vi "sc_decode.vi"(1 "SC_bits":dbl[](array[numeric])) -> (0 "Place opened":string)   [LabVIEW 2017]
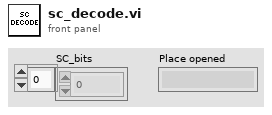
[diagram p1: front panel]
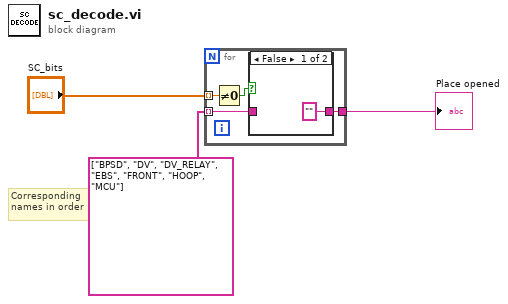
[diagram p0: block diagram]
diagram:
  # "Corresponding names in order"
  n1 = for {
    tunnel: "SC_bits" -> [w7] mode=indexing
    tunnel: string[] ["BPSD", "DV", "DV_RELAY", "EBS", "FRONT", "HOOP", "MCU"] -> [w5] mode=indexing
    tunnel: [w4] -> w3
    n2 = Not Equal To 0?(x=w7) -> (x != 0?=w6:bool)
    n3 = case shown="False" w6 {
      tunnel: w5 -> [_ w9]
      tunnel: ["" ("String") w9] -> w4
      frame False {
      }
      frame True {
      }
    }
  }
  "Place opened" <- w3
